vi "Join Strings.vi"(10 "Delimeter (\", \")":string=", ", 11 "Strings":string[](array[string])) -> (3 "Joined string":string)   [LabVIEW 2010]
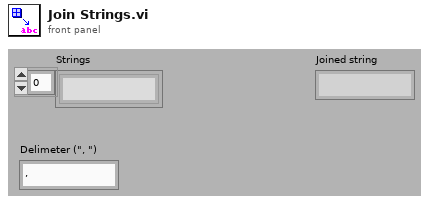
[diagram p1: front panel]
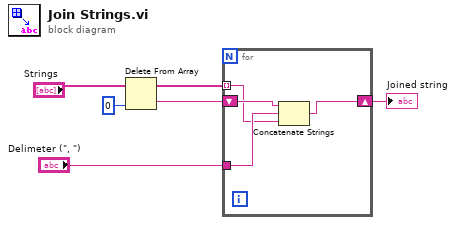
[diagram p0: block diagram]
diagram:
  n1 = Delete From Array(array="Strings", index=0) -> (deleted portion=w5:string, array with subset deleted=w3:string[])  [unwired: 1 in]
  n2 = for {
    shift-right: [w7] -> w2
    shift-left: w5 -> [w10]
    tunnel: "Delimeter (\", \")" -> [w9]
    tunnel: w3 -> [w8] mode=indexing
    n3 = Concatenate Strings(w10, w9, w8) -> (w7:string)
  }
  "Joined string" <- w2
